vi "_PC_Pub_fill_ctrl_panel.vi"(7 "fill_ctrl_ID":u32[](array[numeric])=[8, 15], 8 "error in (no error)":errorcluster, 11 "panel_reference_array":refnum<vi>[](array[refnum])) -> (0 "error out":errorcluster)   [LabVIEW 2018]
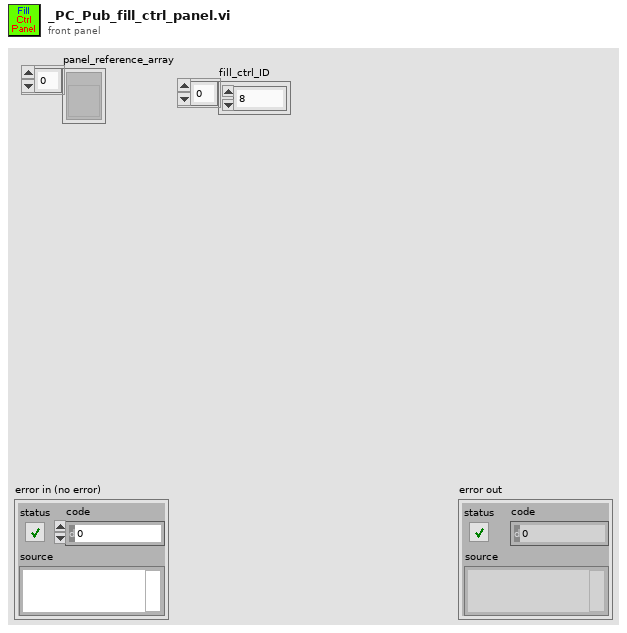
[diagram p1: front panel]
types:
  T1 = enum16{"No Scaling", "Scale All Objects", "Scale Single Object"}
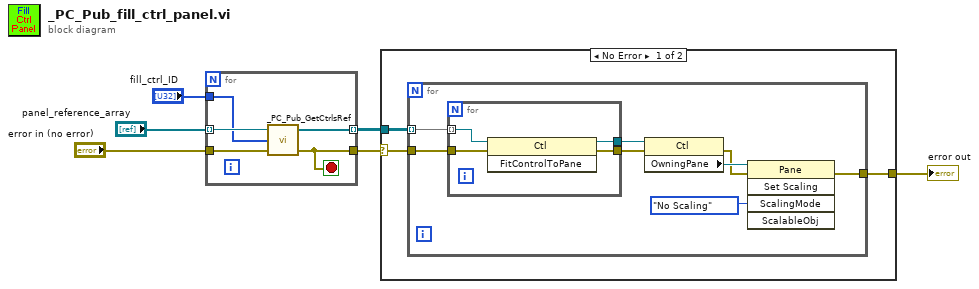
[diagram p0: block diagram]
diagram:
  n1 = for {
    tunnel: "panel_reference_array" -> [w11] mode=indexing
    tunnel: "error in (no error)" -> [w10]
    tunnel: [w7] -> w2
    tunnel: [w9] -> w5 mode=indexing
    tunnel: "fill_ctrl_ID" -> [w8]
    stop <- w7 stop-if-true
    n2 = call "_PC_Pub_GetCtrlsRef.vi"("error in (no error)"=w10, "Ctrls ID"=w8, "Panel Ref"=w11) -> ("error out"=w7:errorcluster, "Ctl Ref Array"=w9:refnum<vi>[])  [unwired: 1 in]
  }
  n3 = case shown="No Error" w2 {
    selector: w2 -> [w12 w27]
    tunnel: w5 -> [w14 _]
    tunnel: [w13 w27] -> w3
    frame No Error {
      n4 = for {
        tunnel: w14 -> [w22] mode=indexing
        tunnel: w12 -> [w21]
        tunnel: [w15] -> w13
        n5 = for {
          tunnel: w22 -> [w24] mode=indexing
          tunnel: w21 -> [w23]
          tunnel: [w26] -> w17
          tunnel: [w25] -> w16
          n6 = invoke class="Ctl" method="FitControlToPane"(reference=w24, error in=w23) -> (reference out=w26:refnum<vi>, error out=w25:errorcluster)  [unwired: 1 in, 1 out]
        }
        n7 = property class="Ctl"(reference=w17, error in=w16) -> (error out=w18:errorcluster, "OwningPane"=w20:refnum<vi>)  [unwired: 1 out]
        n8 = invoke class="Pane" method="Set Scaling"(reference=w20, error in=w18, "ScalingMode"=T1."No Scaling" ("Scaling Mode")) -> (error out=w15:errorcluster)  [unwired: 2 in, 4 out]
      }
    }
    frame Error {
    }
  }
  "error out" <- w3
